vi "FTW-Container-Construct-IR.vi"(5 "Data":variant, 11 "error in":errorcluster) -> (4 "Container":refnum<class "FTW-Container.lvclass">, 6 "Container IR":string, 15 "error out":errorcluster)   [LabVIEW 2012, in "FTW-Container.lvclass"]
uses:
  FTW-Container.lvclass
  <resource>/objmgr/DOMUserDefRef.rc
panel:
  # "Inputs"
  # "Outputs"
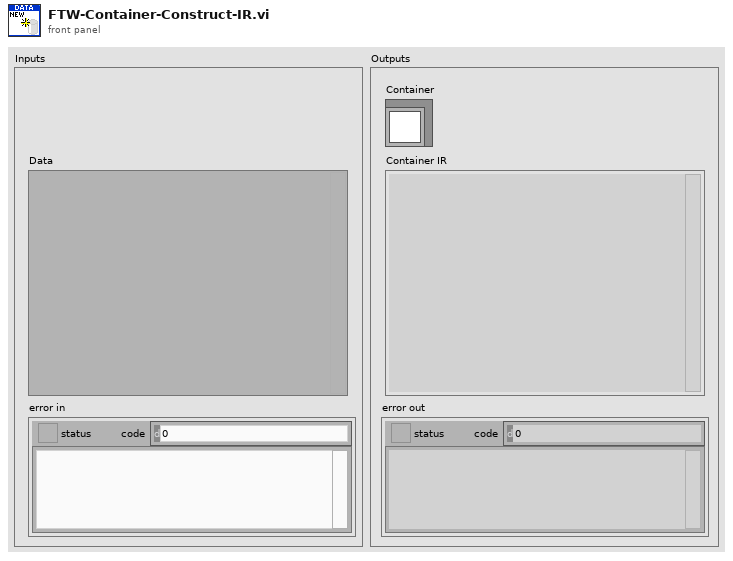
[diagram p1: front panel]
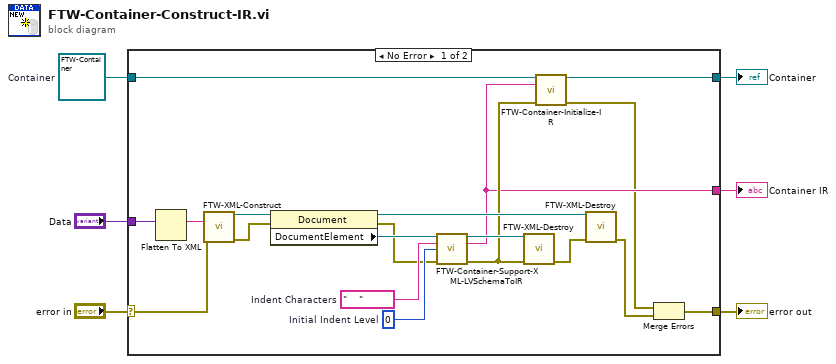
[diagram p0: block diagram]
diagram:
  w3 = refnum<class "FTW-Container.lvclass"> refnum  # Container
  n1 = case shown="No Error" "error in" {
    selector: "error in" -> [w23 w27]
    tunnel: [w21 w27] -> w6
    tunnel: [w10 w26] -> w4
    tunnel: w3 -> [w11 w26]
    tunnel: "Data" -> [w24 _]
    tunnel: [w8 _] -> w1
    frame No Error {
      w19 = 0  # Initial Indent Level
      w20 = "    "  # Indent Characters
      n2 = Flatten To XML(anything=w24) -> (xml string=w25:string)
      n3 = call "FTW-XML-Construct.vi"("XML String"=w25, "error in"=w23) -> ("XML Document"=w18:refnum<k20>, "error out"=w16:errorcluster)  [unwired: 12 in]
      n4 = property class="Document"(reference=w18, error in=w16) -> (reference out=w14:refnum<k20>, error out=w15:errorcluster, "DocumentElement"=w17:refnum<k20>)
      n5 = call "FTW-Container-Support-XML-LVSchemaToIR.vi"("XML Node"=w17, "Indent Characters"=w20, "Indent Level"=w19, "error in"=w15) -> ("XML Node out"=w22:refnum<k20>, "Serialized Node"=w8:string, "error out"=w9:errorcluster)  [unwired: 9 in]
      n6 = call "FTW-XML-Destroy.vi"("XML Node"=w22, "error in"=w9) -> ("error out"=w13:errorcluster)  [unwired: 13 in]
      n7 = call-dynamic "FTW-Container-Initialize-IR.vi"("Container"=w11, "Container IR"=w8, "error in"=w9) -> ("Container out"=w10:refnum<class "FTW-Container.lvclass">, "error out"=w7:errorcluster)  [unwired: 11 in]
      n8 = call "FTW-XML-Destroy.vi"("XML Node"=w14, "error in"=w13) -> ("error out"=w12:errorcluster)  [unwired: 13 in]
      n9 = Merge Errors(w7, w12) -> (w21:errorcluster)
    }
    frame Error {
    }
  }
  "error out" <- w6
  "Container" <- w4
  "Container IR" <- w1
